vi "TemplateUI.vi"() -> ()   [LabVIEW 2016]
uses:
  Package ResourceControl/ViHandler/ViHandler.ViInfo.ctl
  Message Queue/private/MessageQueue.MessageTypeDef.ctl
  Package ResourceControl/ViHandler/ViHandler.RunModes.ctl
  Package ErrorHandling/ErrorHandling.lvclass/ErrorHandling.ctl
  Package ErrorHandling/ErrorHandling.checkForErrorAndHandle.vi
  Package ErrorHandling/ErrorHandling.GetErrorHandler.vi
  <vilib>/Utility/error.llb/Clear Errors.vi
  StringFunctions/StringFunctions_ReplaceAllBlindSigns.vi
  <vilib>/dlg_ctls.llb/Space Constant.vi
  <vilib>/Utility/error.llb/Error Cluster From Error Code.vi
  TimingFunctions/TimingFunctions_getUtcTimestamp.vi
  <vilib>/Utility/error.llb/Trim Whitespace.vi
  <vilib>/Utility/error.llb/Search and Replace Pattern.vi
  Package ErrorHandling/ErrorHandling.addLastErrorToFile.vi
  <vilib>/ErrorRing/Error Ring.xnode
  Package ErrorHandling/ErrorHandling.lvclass
panel:
  out "LoadedPanel":enum16{"Button1", "Button2", "Button3"}(ring)
  in  "Button3Btn":bool
  out "Exp.StorageName":string
  out "ViInfoTemp":T1
  in  "Button2Btn":bool
  in  "Button1Btn":bool
  # "Please chose the desired conversion method"
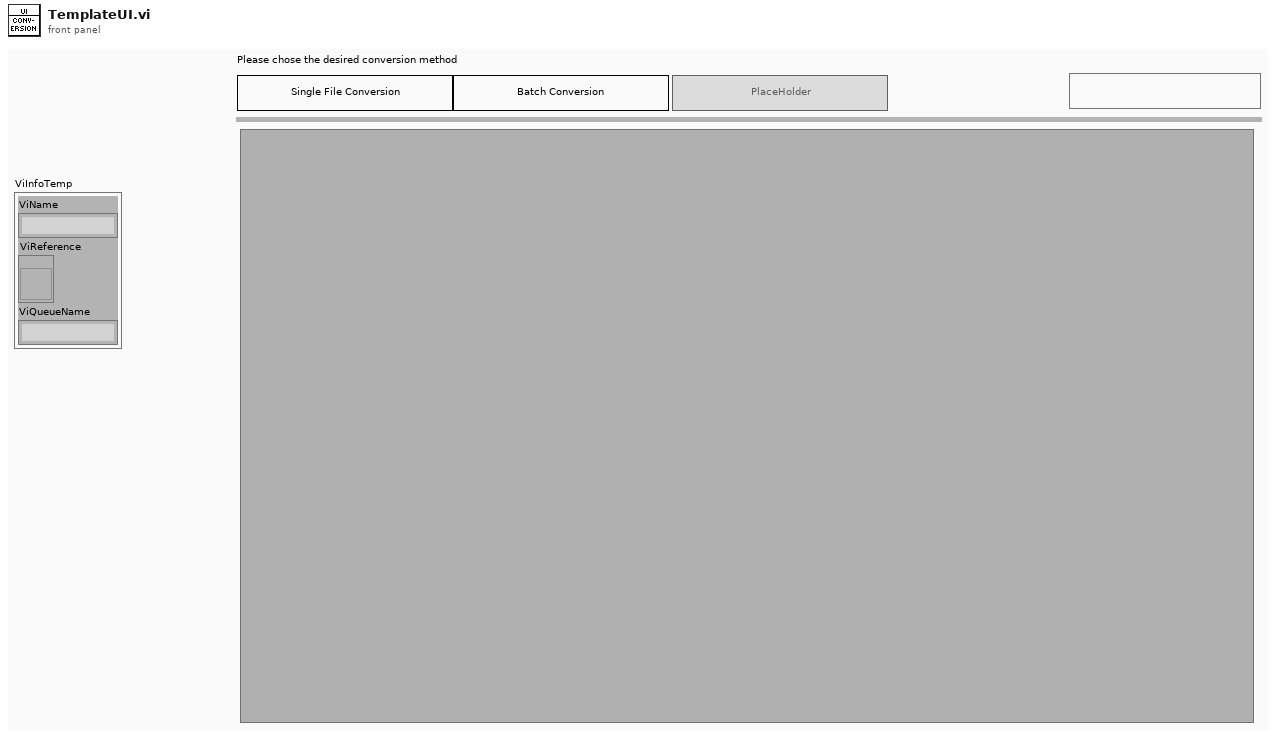
[diagram p1: front panel]
types:
  T1 = typedef "ViHandler.lvclass/ViHandler.ViInfo.ctl" = cluster{"ViName":string, "ViReference":refnum<vi>, "ViQueueName":string}
  T2 = typedef "MessageQueue.MessageTypeDef.ctl" = cluster{"Message":string, "Data":variant}
  T3 = typedef "ViHandler.lvclass/ViHandler.RunModes.ctl" = enum16{"FP Closed", "FP Open", "FP Open, Centered"}
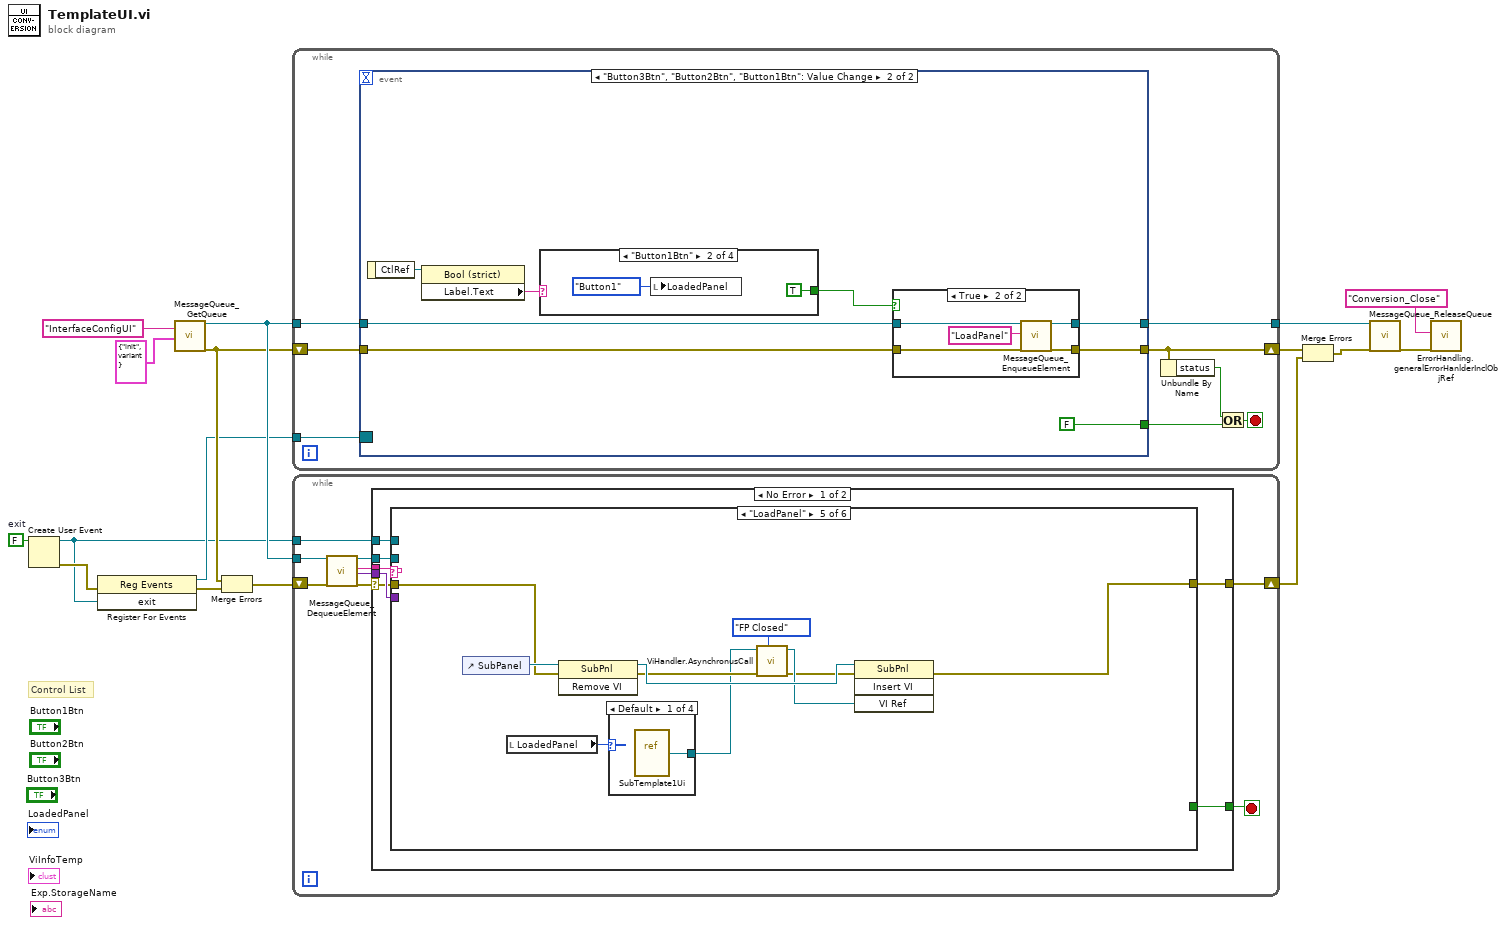
[diagram p0: block diagram]
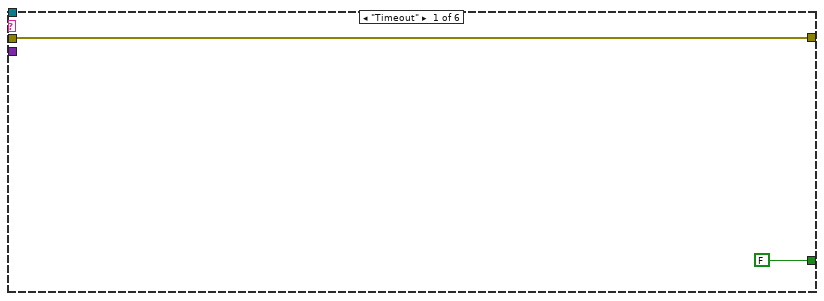
[diagram p2: hidden frame]
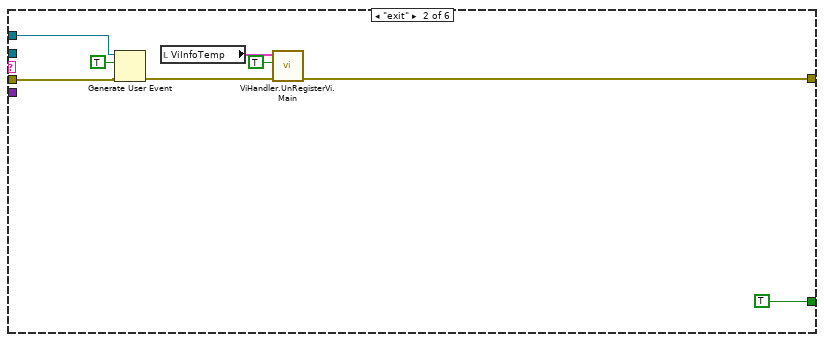
[diagram p3: hidden frame]
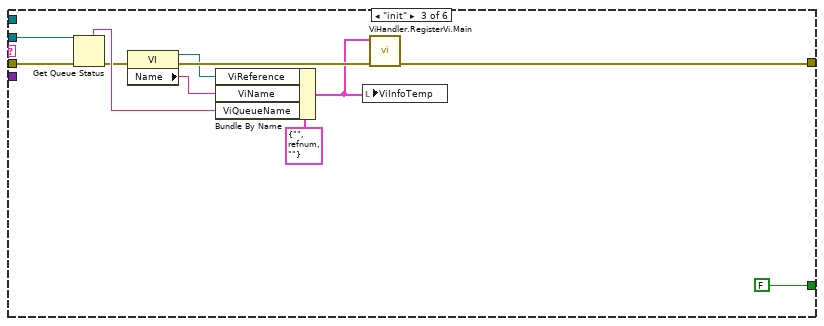
[diagram p4: hidden frame]
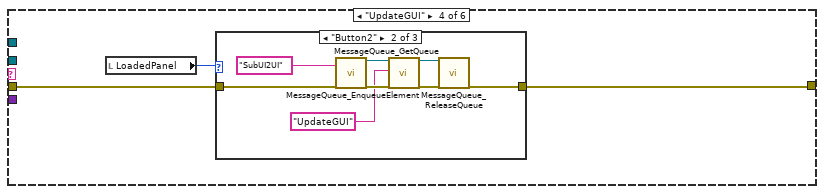
[diagram p5: hidden frame]
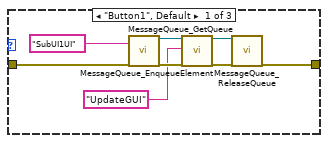
[diagram p6: hidden frame]
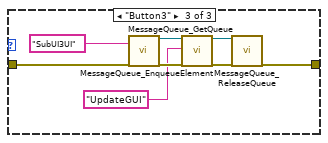
[diagram p7: hidden frame]
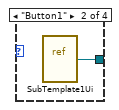
[diagram p8: hidden frame]
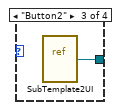
[diagram p9: hidden frame]
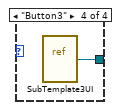
[diagram p10: hidden frame]
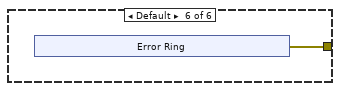
[diagram p11: hidden frame]
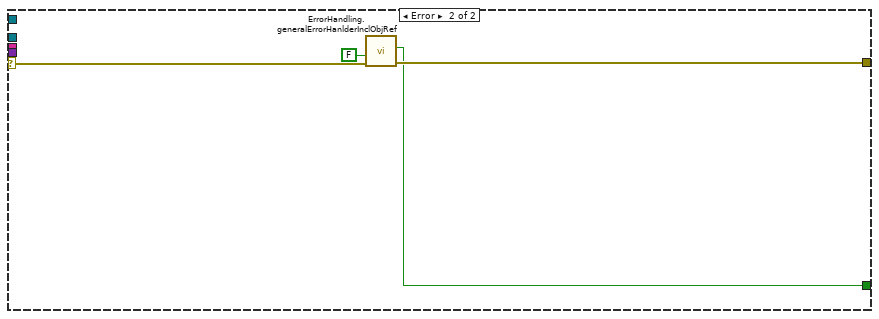
[diagram p12: hidden frame]
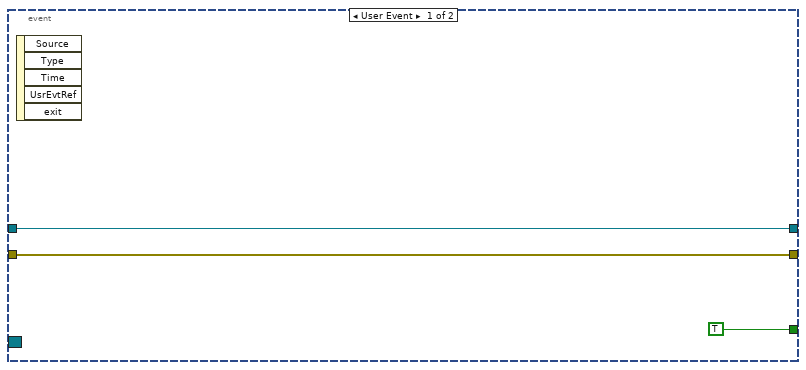
[diagram p13: hidden frame]
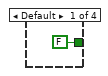
[diagram p15: hidden frame]
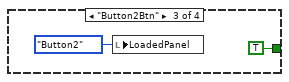
[diagram p16: hidden frame]
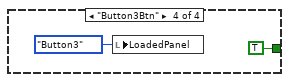
[diagram p17: hidden frame]
diagram:
  w9 = FALSE  # exit
  # "Control List"
  n1 = Create User Event(user event datatype=w9) -> (user event=w7:refnum<user-event>, error out=w8:errorcluster)  [unwired: 1 in]
  n2 = register-events(error in=w8, w7) -> (reference out=w11:refnum<event-registration>, error out=w13:errorcluster)  [unwired: 1 in]
  n3 = call "MessageQueue_GetQueue.vi"("Name"="InterfaceConfigUI", "OptionalInitValue"=T2 {"Message"="init", "Data"=variant}) -> ("QueueOut"=w15:refnum<queue>, "ErrorOut"=w12:errorcluster)  [unwired: 15 in, 1 out]
  n4 = Merge Errors(w12, w13) -> (w10:errorcluster)
  n5 = while {
    tunnel: w15 -> [w24]
    tunnel: [w23] -> w16
    shift-right: [w20] -> w5
    shift-left: w12 -> [w22]
    tunnel: w11 -> [w17]
    stop <- w19 stop-if-true
    n6 = event shown="[1] \"Button3Btn\", \"Button2Btn\", \"Button1Btn\": Value Change" {
      selector: w17 -> [_ _]
      dyn-events: _ -> [_ _]
      timeout: _ -> [_ _]
      tunnel: w24 -> [w26 w35]
      tunnel: [w26 w34] -> w23
      tunnel: [w25 w33] -> w20
      tunnel: w22 -> [w25 w32]
      tunnel: [TRUE FALSE] -> w21
      event User Event {
        n7 = event-data() -> ()  [unwired: 1 in, 5 out]
      }
      event "Button3Btn", "Button2Btn", "Button1Btn": Value Change {
        n8 = event-data() -> ("CtlRef"=w30:refnum<vi>)  [unwired: 1 in]
        n9 = property class="Bool (strict)"(reference=w30) -> ("Label.Text"=w29:string)  [unwired: 1 in, 2 out]
        n10 = case shown="\"Button1Btn\"" w29 {
          tunnel: [FALSE TRUE TRUE TRUE] -> w28
          frame Default {
          }
          frame "Button1Btn" {
            n11 = local write "LoadedPanel"(enum16{"Button1", "Button2", "Button3"}."Button1") -> ()
          }
          frame "Button2Btn" {
            n12 = local write "LoadedPanel"(enum16{"Button1", "Button2", "Button3"}."Button2") -> ()
          }
          frame "Button3Btn" {
            n13 = local write "LoadedPanel"(enum16{"Button1", "Button2", "Button3"}."Button3") -> ()
          }
        }
        n14 = case shown="True" w28 {
          tunnel: w35 -> [w37 w42]
          tunnel: [w37 w41] -> w34
          tunnel: [w36 w40] -> w33
          tunnel: w32 -> [w36 w39]
          frame False {
          }
          frame True {
            n15 = call "MessageQueue_EnqueueElement.vi"("QueueIn"=w42, "Message"="LoadPanel", "ErrorIn"=w39) -> ("QueueOut"=w41:refnum<queue>, "ErrorOut"=w40:errorcluster)  [unwired: 15 in]
          }
        }
      }
    }
    n16 = Unbundle By Name(w20) -> ("status"=w18:bool)
    n17 = Or(x=w18, y=w21) -> (x .or. y?=w19:bool)
  }
  n18 = while {
    tunnel: w15 -> [w58]
    tunnel: w7 -> [w51]
    shift-right: [w50] -> w4
    shift-left: w10 -> [w52]
    stop <- w53 stop-if-true
    n19 = call "MessageQueue_DequeueElement.vi"("QueueIn"=w58, "ErrorIn"=w52) -> ("QueueOut"=w56:refnum<queue>, "Message"=w55:string, "Data"=w54:variant, "ErrorOut"=w57:errorcluster)  [unwired: 13 in, 1 out]
    n20 = case shown="No Error" w57 {
      selector: w57 -> [w61 w137]
      tunnel: w56 -> [w65 _]
      tunnel: w55 -> [w64 _]
      tunnel: w54 -> [w63 _]
      tunnel: [w62 w134] -> w53
      tunnel: w51 -> [w60 _]
      tunnel: [w59 w136] -> w50
      frame No Error {
        n21 = case shown="\"LoadPanel\"" w64 {
          tunnel: w65 -> [_ _ w78 _ _ _]
          tunnel: w63 -> [_ _ _ _ _ _]
          tunnel: [FALSE TRUE FALSE _ _ _] -> w62
          tunnel: w61 -> [w66 w73 w79 w89 w116 _]
          tunnel: w60 -> [_ w72 _ _ _ _]
          tunnel: [w66 w69 w77 w88 w115 w128] -> w59
          frame "Timeout" {
          }
          frame "exit" {
            n22 = Generate User Event(user event=w72, event data cluster=TRUE ("event data"), error in=w73) -> (error out=w70:errorcluster)  [unwired: 1 in, 1 out]
            n23 = local read "ViInfoTemp"() -> (w71:T1)
            n24 = call "ViHandler.UnRegisterVi.Main.vi"("ErrorIn"=w70, "FinalExit?"=TRUE, "ViInfo"=w71) -> ("ErrorOut"=w69:errorcluster)  [unwired: 7 in, 1 out]
          }
          frame "init" {
            n25 = Get Queue Status(queue=w78, error in (no error)=w79) -> (queue name=w84:string, error out=w83:errorcluster)  [unwired: 1 in, 6 out]
            n26 = property class="VI"(error in=w83) -> (reference out=w81:refnum<vi>, error out=w82:errorcluster, "Name"=w80:string)  [unwired: 1 in]
            n27 = Bundle By Name(cluster=T1 {"ViName"="", "ViReference"=refnum, "ViQueueName"=""} ("ViInfo"), "ViReference"=w81, "ViName"=w80, "ViQueueName"=w84) -> (w76:T1)
            n28 = local write "ViInfoTemp"(w76) -> ()
            n29 = call "ViHandler.RegisterVi.Main.vi"("ErrorIn"=w82, "ViInfo"=w76) -> ("ErrorOut"=w77:errorcluster)  [unwired: 9 in]
          }
          frame "UpdateGUI" {
            n30 = local read "LoadedPanel"() -> (w87:enum16{"Button1", "Button2", "Button3"})
            n31 = case shown="\"Button2\"" w87 {
              tunnel: w89 -> [w97 w105 w113]
              tunnel: [w92 w100 w108] -> w88
              frame "Button1", Default {
                n32 = call "MessageQueue_GetQueue.vi"("Name"="SubUI1UI", "ErrorIn"=w97) -> ("QueueOut"=w94:refnum<queue>, "ErrorOut"=w96:errorcluster)  [unwired: 15 in, 1 out]
                n33 = call "MessageQueue_EnqueueElement.vi"("QueueIn"=w94, "Message"="UpdateGUI", "ErrorIn"=w96) -> ("QueueOut"=w95:refnum<queue>, "ErrorOut"=w93:errorcluster)  [unwired: 15 in]
                n34 = call "MessageQueue_ReleaseQueue.vi"("QueueIn"=w95, "ErrorIn"=w93) -> ("ErrorOut"=w92:errorcluster)  [unwired: 15 in, 2 out]
              }
              frame "Button2" {
                n35 = call "MessageQueue_GetQueue.vi"("Name"="SubUI2UI", "ErrorIn"=w105) -> ("QueueOut"=w102:refnum<queue>, "ErrorOut"=w104:errorcluster)  [unwired: 15 in, 1 out]
                n36 = call "MessageQueue_EnqueueElement.vi"("QueueIn"=w102, "Message"="UpdateGUI", "ErrorIn"=w104) -> ("QueueOut"=w103:refnum<queue>, "ErrorOut"=w101:errorcluster)  [unwired: 15 in]
                n37 = call "MessageQueue_ReleaseQueue.vi"("QueueIn"=w103, "ErrorIn"=w101) -> ("ErrorOut"=w100:errorcluster)  [unwired: 15 in, 2 out]
              }
              frame "Button3" {
                n38 = call "MessageQueue_GetQueue.vi"("Name"="SubUI3UI", "ErrorIn"=w113) -> ("QueueOut"=w110:refnum<queue>, "ErrorOut"=w112:errorcluster)  [unwired: 15 in, 1 out]
                n39 = call "MessageQueue_EnqueueElement.vi"("QueueIn"=w110, "Message"="UpdateGUI", "ErrorIn"=w112) -> ("QueueOut"=w111:refnum<queue>, "ErrorOut"=w109:errorcluster)  [unwired: 15 in]
                n40 = call "MessageQueue_ReleaseQueue.vi"("QueueIn"=w111, "ErrorIn"=w109) -> ("ErrorOut"=w108:errorcluster)  [unwired: 15 in, 2 out]
              }
            }
          }
          frame "LoadPanel" {
            n41 = control-ref of="SubPanel"() -> (w117:refnum<vi>)
            n42 = local read "LoadedPanel"() -> (w114:enum16{"Button1", "Button2", "Button3"})
            n43 = invoke on="Invoke Node" class="SubPnl" method="Remove VI"(reference=w117, error in=w116) -> (reference out=w123:refnum<vi>, error out=w119:errorcluster)  [unwired: 1 in, 1 out]
            n44 = case shown="Default" w114 {
              tunnel: [w124 w125 w126 w127] -> w118
              frame Default {
                n45 = vi-ref "SubTemplate1Ui.vi"() -> (w124:refnum<vi>)
              }
              frame "Button1" {
                n46 = vi-ref "SubTemplate1Ui.vi"() -> (w125:refnum<vi>)
              }
              frame "Button2" {
                n47 = vi-ref "SubTemplate2UI.vi"() -> (w126:refnum<vi>)
              }
              frame "Button3" {
                n48 = vi-ref "SubTemplate3UI.vi"() -> (w127:refnum<vi>)
              }
            }
            n49 = call "ViHandler.AsynchronusCall.vi"("Modes"=ViHandler.RunModes."FP Closed", "Error In"=w119, "ViReference"=w118) -> ("error out"=w120:errorcluster, "ViReference"=w121:refnum<vi>)  [unwired: 5 in, 2 out]
            n50 = invoke on="Invoke Node" class="SubPnl" method="Insert VI"(reference=w123, error in=w120, "VI Ref"=w121) -> (error out=w115:errorcluster)  [unwired: 1 in, 3 out]
          }
          frame Default {
            n51 = xnode "Error Ring"() -> ("error out"=w128:errorcluster)
          }
        }
      }
      frame Error {
        n52 = call "ErrorHandling.generalErrorHanlderInclObjRef.vi"("error in"=w137, "StopOnError"=FALSE) -> ("error out"=w136:errorcluster, "Stop"=w134:bool)  [unwired: 7 in, 1 out]
      }
    }
  }
  n53 = Merge Errors(w5, w4) -> (w3:errorcluster)
  n54 = call "MessageQueue_ReleaseQueue.vi"("QueueIn"=w16, "ErrorIn"=w3) -> ("ErrorOut"=w2:errorcluster)  [unwired: 15 in, 2 out]
  n55 = call "ErrorHandling.generalErrorHanlderInclObjRef.vi"("error in"=w2, "Comment(optional)"="Conversion_Close") -> ()  [unwired: 7 in, 3 out]
